vi "GetMacAddress.vi"() -> ()   [LabVIEW 2012]
panel:
  out "Mac Address":string
  out "standard output":string
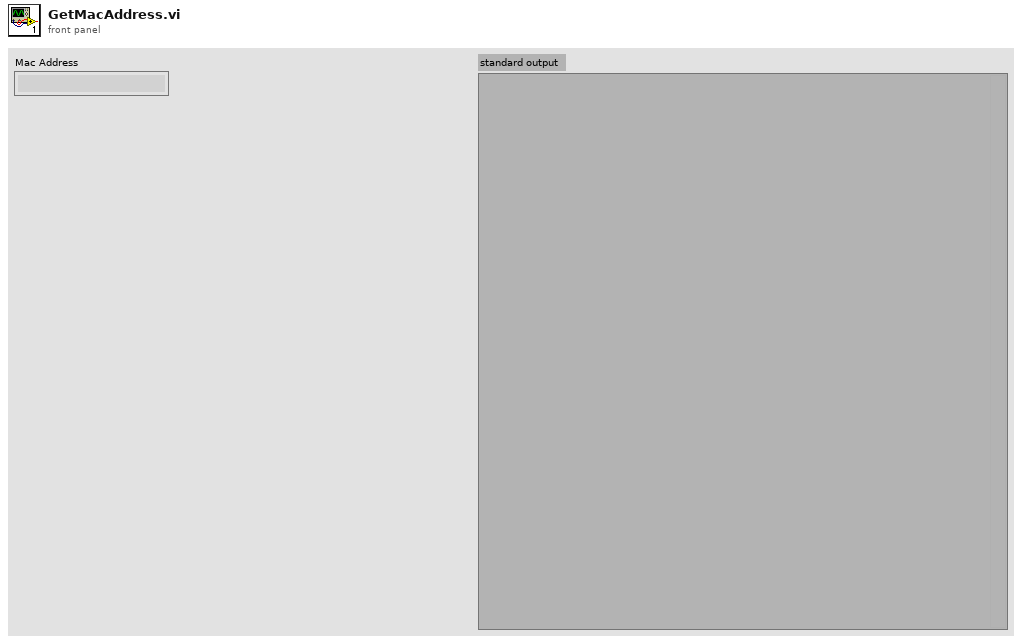
[diagram p1: front panel]
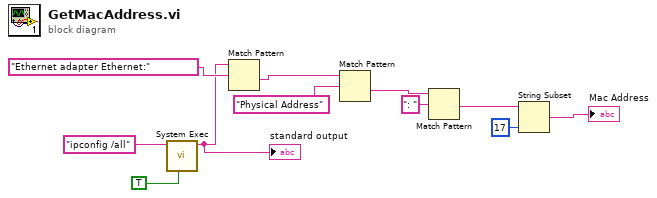
[diagram p0: block diagram]
diagram:
  n1 = call <vilib>:"System Exec.vi"("run minimized? (F)"=TRUE, "command line"="ipconfig /all") -> ("standard output"=w8:string)  [unwired: 6 in, 3 out]
  "standard output" <- w8
  n2 = Match Pattern(string=w8, regular expression="Ethernet adapter Ethernet:" ("string")) -> (after substring=w7:string)  [unwired: 1 in, 3 out]
  n3 = Match Pattern(string=w7, regular expression="Physical Address") -> (after substring=w5:string)  [unwired: 1 in, 3 out]
  n4 = Match Pattern(string=w5, regular expression=": ") -> (after substring=w3:string)  [unwired: 1 in, 3 out]
  n5 = String Subset(string=w3, length (rest)=17 ("length (rest)")) -> (substring=→"Mac Address":string)  [unwired: 1 in]
